vi "retrieveDeviceInformation.vi"(8 "error in (no error)":errorcluster, 11 "TEI9150 in":refnum<class "TEI9150.lvclass">) -> (0 "error out":errorcluster, 2 "Device Information":string, 3 "TEI9150 out":refnum<class "TEI9150.lvclass">)   [LabVIEW 2015, in "TEI9150.lvclass"]
uses:
  TEI9150.lvclass
  TEI9150.lvclass/TEI9150.ctl
  <userlib>/Common/SerialProtocols/SerialCommunicator/SerialCommunicator.lvclass
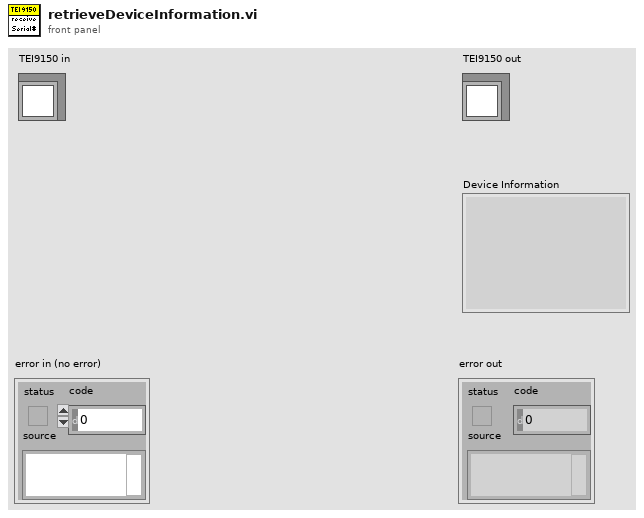
[diagram p1: front panel]
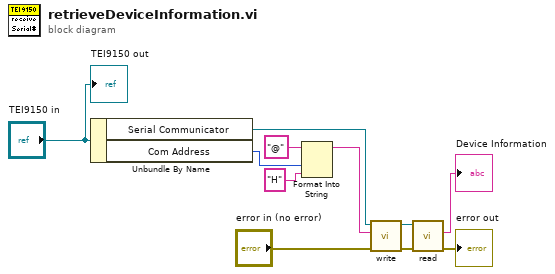
[diagram p0: block diagram]
diagram:
  n1 = Unbundle By Name("TEI9150 in") -> ("Serial Communicator"=w11:refnum<class "SerialCommunicator.lvclass">, "Com Address"=w9:u8)
  n2 = Format Into String(initial string="@" ("string"), w9, "H" ("string")) -> (resulting string=w7:string)  [unwired: 2 in, 1 out]
  n3 = call-dynamic "write.vi"("error in (no error)"="error in (no error)", "writeString"=w7, "SerialCommunicator in"=w11) -> ("error out"=w4:errorcluster, "SerialCommunicator out"=w6:refnum<class "SerialCommunicator.lvclass">)  [unwired: 7 in]
  n4 = call-dynamic "read.vi"("error in (no error)"=w4, "SerialCommunicator in"=w6) -> ("error out"=→"error out":errorcluster, "stringRead"=→"Device Information":string)  [unwired: 7 in, 1 out]
  "TEI9150 out" <- "TEI9150 in"
